vi "controller8.vi"(8 "Neg max speed":dbl=-1.0, 10 "reverse":bool, 11 "obs":bool) -> ()   [LabVIEW 2015]
uses:
  G_ALL.vi
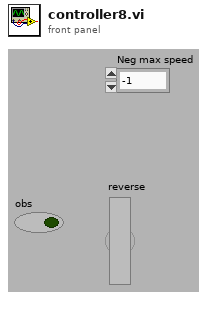
[diagram p1: front panel]
types:
  T1 = cluster{"Steer_input":dbl, "Steer_output":dbl, "VS_des":dbl, "VS_can":dbl, "heading":dbl, "auto":bool, "run":bool, "x":dbl, "y":dbl}
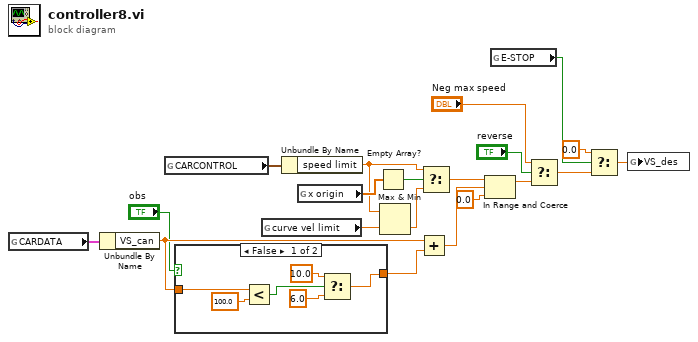
[diagram p0: block diagram]
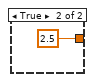
[diagram p2: hidden frame]
diagram:
  n1 = global read "G_ALL.vi" "CARDATA"() -> (w7:T1)
  n2 = Unbundle By Name(w7) -> ("VS_can"=w10:dbl)
  n3 = global read "G_ALL.vi" "CARCONTROL"() -> (w14:cluster{"speed path":dbl, "speed limit":dbl})
  n4 = case shown="False" "obs" {
    tunnel: w10 -> [w26 _]
    tunnel: [w25 2.5 ("upper limit")] -> w9
    frame False {
      n5 = Less?(x=w26, y=100.0) -> (x < y?=w23:bool)
      n6 = Select(t=10.0 ("upper limit"), s=w23, f=6.0 ("upper limit")) -> (s? t:f=w25:dbl)
    }
    frame True {
    }
  }
  n7 = global read "G_ALL.vi" "curve vel limit"() -> (w12:dbl)
  n8 = Unbundle By Name(w14) -> ("speed limit"=w4:dbl)
  n9 = global read "G_ALL.vi" "x origin"() -> (w6:dbl[])
  n10 = Empty Array?(array=w6) -> (empty?=w5:bool)
  n11 = Max & Min(x=w4, y=w12) -> (min(x,y)=w2:dbl)  [unwired: 1 out]
  n12 = Add(x=w10, y=w9) -> (x+y=w16:dbl)
  n13 = Select(t=w4, s=w5, f=w2) -> (s? t:f=w3:dbl)
  n14 = In Range and Coerce(upper limit=w3, x=w16, lower limit=0.0) -> (coerced(x)=w1:dbl)  [unwired: 1 out]
  n15 = global read "G_ALL.vi" "E-STOP"() -> (w15:bool)
  n16 = Select(t="Neg max speed", s="reverse", f=w1) -> (s? t:f=w11:dbl)
  n17 = Select(t=0.0, s=w15, f=w11) -> (s? t:f=w13:dbl)
  n18 = global write "G_ALL.vi" "VS_des"(w13) -> ()
